vi "Periodic Tasks.vi"(8 "error in":errorcluster) -> ()   [LabVIEW 2013]
doc: "This VI runs in parallel to other tasks. It can contain as many user-defined periodic loops as you need. These can carry out PID or other sorts of timed response."
uses:
  <vilib>/Rock Robotics/WPI/Compressor/WPI_CompressorDevRef.ctl
  <vilib>/Rock Robotics/WPI/DigitalInput/WPI_DigitalInputDevRef.ctl
  <vilib>/Rock Robotics/SystemInterfaces/DIO/FPGA_DIOChannel.ctl
  <vilib>/Rock Robotics/SystemInterfaces/Typedef/FPGA_TypedefDigitalModule.ctl
  <vilib>/Rock Robotics/WPI/Relay/WPI_RelayDevRef.ctl
  <vilib>/Rock Robotics/SystemInterfaces/DIO/FPGA_DIORelayChannel.ctl
  <vilib>/Rock Robotics/WPI/Relay/WPI_RelayDirection.ctl
  <vilib>/Rock Robotics/SystemInterfaces/Utilities/FPGA_UtilitiesLED Source.ctl
  <vilib>/Rock Robotics/SystemInterfaces/Utilities/FPGA_UtilitiesLED State.ctl
  <vilib>/Rock Robotics/WPI/RobotDrive/WPI_RobotDriveGetSetRefNum.vi
  Robot Global Data.vi
  <vilib>/Rock Robotics/WPI/Joystick/WPI_JoystickGetSetRefNum.vi
panel:
  out "output cluster":T1={"DevStatus"={"status"=FALSE, "code"=0, "source"=""}, "DigitalInputDevRef"={"DevStatus"={"status"=FALSE, "code"=0, "source"=""}, "DIO Channel"=enum."DIO 1", "Digital Module"=enum."Digital Module 1"}, "RelayDevRef"={"DevStatus"={"status"=FALSE, "code"=0, "source"=""}, "Relay Channel"=enum."Invalid", "Digital Module"=enum."Digital Module 1", "Relay Direction"=enum."Both directions"}}
  out "Robot Driving":bool
  out "10 ms Counter":i32
  out "100 ms Counter":i32
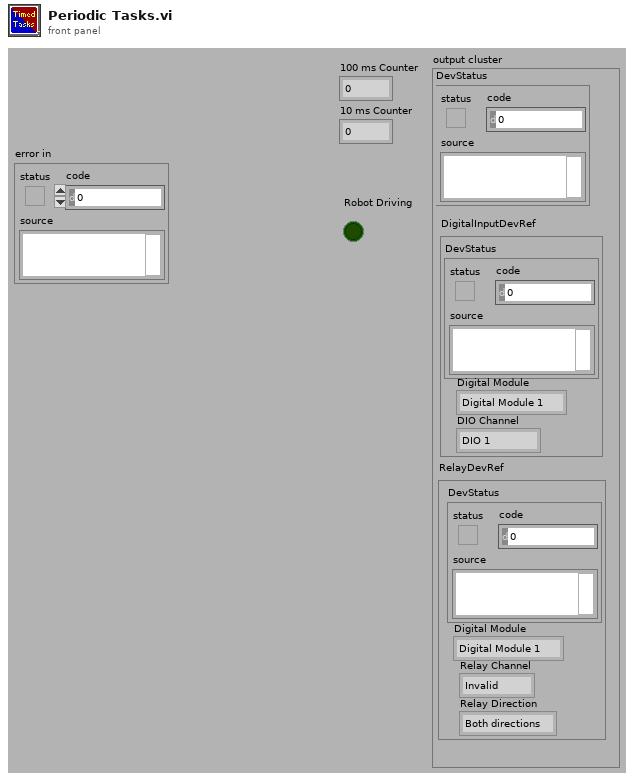
[diagram p1: front panel]
types:
  T1 = typedef "WPI_CompressorDevRef.ctl" = cluster{"DevStatus":errorcluster, "DigitalInputDevRef":T2, "RelayDevRef":T5}
  T2 = typedef "WPI_DigitalInputDevRef.ctl" = cluster{"DevStatus":errorcluster, "DIO Channel":T3, "Digital Module":T4}
  T3 = typedef "FPGA_DIOChannel.ctl" = enum8{"DIO 1", "DIO 2", "DIO 3", "DIO 4", "DIO 5", "DIO 6", "DIO 7", "DIO 8", "DIO 9", "DIO 10", "DIO 11", "DIO 12", "DIO 13", "DIO 14", "Invalid"}
  T4 = typedef "FPGA_TypedefDigitalModule.ctl" = enum16{"Digital Module 1", "Digital Module 2"}
  T5 = typedef "WPI_RelayDevRef.ctl" = cluster{"DevStatus":errorcluster, "Relay Channel":T6, "Digital Module":T4, "Relay Direction":T7}
  T6 = typedef "FPGA_DIORelayChannel.ctl" = enum8{"Relay 1", "Relay 2", "Relay 3", "Relay 4", "Relay 5", "Relay 6", "Relay 7", "Relay 8", "Invalid"}
  T7 = typedef "WPI_RelayDirection.ctl" = enum16{"Both directions", "Forward only", "Reverse only"}
  T8 = typedef "FPGA_UtilitiesLED State.ctl" = enum16{"Off", "On", "Toggle"}
  T9 = typedef "FPGA_UtilitiesLED Source.ctl" = enum16{"User LED", "FPGA LED"}
  T10 = typedef "WPI_JoystickDevRef.ctl" = cluster{"Device":T11}
  T11 = typedef "WPI_JoystickDeviceEnum.ctl" = enum16{"USB 1", "USB 2", "USB 3", "USB 4", "Kinect 1", "Kinect 2"}
  T12 = typedef "WPI_RobotDriveDevRef.ctl" = cluster{"DevStatus":errorcluster, "Motors[]":T13[], "Square Inputs":bool, "Max Output":dbl, "Isochronous":bool}
  T13 = typedef "WPI_MotorControlDeviceRef.ctl" = cluster{"DeviceStatus":errorcluster, "Type":enum16{"PWM", "CAN"}, "PWM":cluster{"Digital Module":T4, "PWM Channel":T14, "DeadBand":T15}, "CAN":cluster{"Device Number":u8, "Control Mode":T16, "Semaphore":T17, "Max Vout":dbl}, "Invert":bool, "TransformRef":T18, "InvTransformRef":T18}
  T14 = typedef "FPGA_DIOPWMChannel.ctl" = enum8{"PWM 1", "PWM 2", "PWM 3", "PWM 4", "PWM 5", "PWM 6", "PWM 7", "PWM 8", "PWM 9", "PWM 10", "Invalid"}
  T15 = typedef "WPI_PWMDeadband.ctl" = cluster{"Name":string, "maxPositivePwm":i32, "minPositivePwm":i32, "centerPwm":i32, "maxNegativePwm":i32, "minNegativePwm":i32, "angularRange":u16}
  T16 = typedef "WPI_CANJaguar_ControlMode.ctl" = enum8{"Percent VBus", "Current", "Speed", "Position", "Voltage"}
  T17 = typedef "Semaphore RefNum" = refnum<k1>
  T18 = typedef "WPI_PWMTransform_ConPane.ctl" = refnum<vi>
  T19 = cluster{"JoystickDevRef":T10, "RobotDriveDevRef":T12}
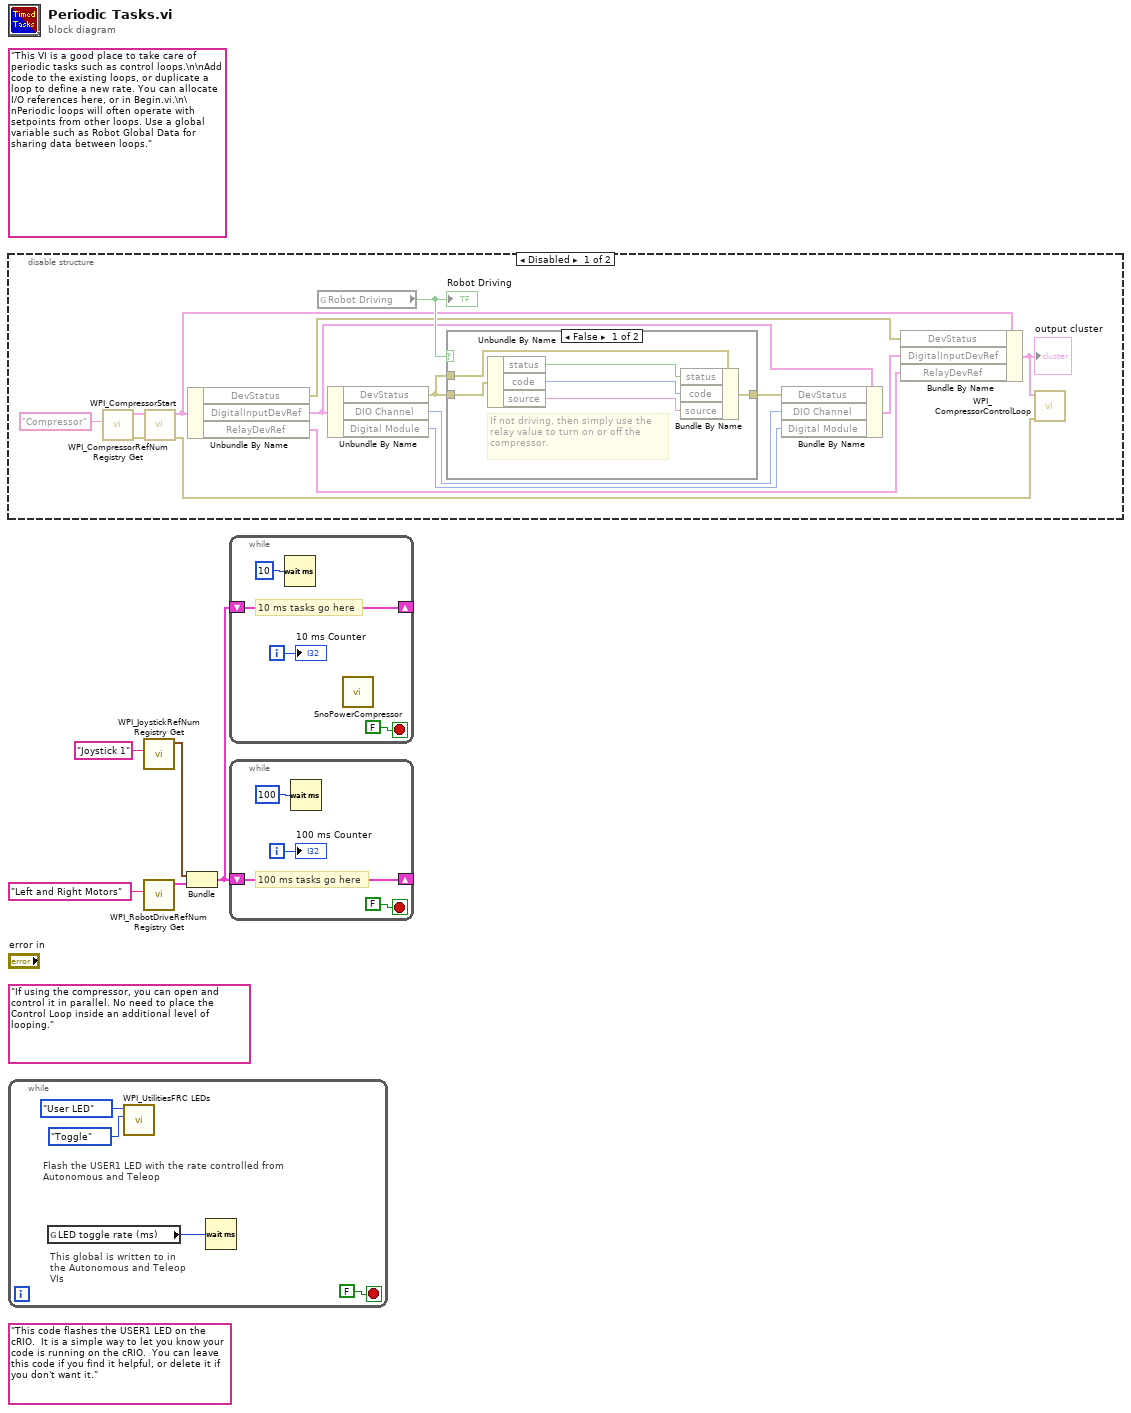
[diagram p0: block diagram]
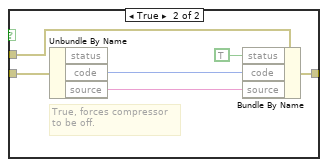
[diagram p2: hidden frame]
diagram:
  (unwired) "If using the compressor, you can open and control it in parallel. No need to place the Control Loop inside an additional level of looping."
  (unwired) "This code flashes the USER1 LED on the cRIO.  It is a simple way to let you know your code is running on the cRIO.  You can leave this code if you find it helpful, or delete it if you don't want it."
  (unwired) "This VI is a good place to take care of periodic tasks such as control loops.\n\nAdd code to the existing loops, or duplicate a loop to define a new rate. You can allocate I/O references here, or in Begin.vi.\n\nPeriodic loops will often operate with setpoints from other loops. Use a global variable such as Robot Global Data for sharing data between loops."
  n1 = disable-structure shown="Disabled" {
    frame Disabled {
      n2 = call <vilib>:"WPI_CompressorRefNum Registry Get.vi"("refnum name"="Compressor") -> ("error out"=w18:errorcluster, "CompressorDevRef"=w19:T1)  [unwired: 9 in]
      n3 = call <vilib>:"WPI_CompressorStart.vi"("error in (no error)"=w18, "CompressorDevRef"=w19) -> ("error out"=w17:errorcluster, "CompressorDevRef"=w12:T1)  [unwired: 8 in]
      n4 = Unbundle By Name(w12) -> ("DevStatus"=w11:errorcluster, "DigitalInputDevRef"=w15:T2, "RelayDevRef"=w10:T5)
      n5 = global read "Robot Global Data.vi" "Robot Driving"() -> (w16:bool)
      "Robot Driving" <- w16
      n6 = Unbundle By Name(w15) -> ("DevStatus"=w7:errorcluster, "DIO Channel"=w14:T3, "Digital Module"=w13:T4)
      n7 = case shown="False" w16 {
        tunnel: [w21 w32] -> w8
        tunnel: w7 -> [w23 w31]
        tunnel: w7 -> [w22 w30]
        frame False {
          # "If not driving, then simply use the\nrelay value to turn on or off the\ncompressor."
          n8 = Unbundle By Name(w22) -> ("status"=w26:bool, "code"=w25:i32, "source"=w24:string)
          n9 = Bundle By Name(cluster=w23, "status"=w26, "code"=w25, "source"=w24) -> (w21:errorcluster)
        }
        frame True {
          # "True, forces compressor\nto be off."
          n10 = Unbundle By Name(w30) -> ("code"=w29:i32, "source"=w28:string)  [unwired: 1 out]
          n11 = Bundle By Name(cluster=w31, "status"=TRUE, "code"=w29, "source"=w28) -> (w32:errorcluster)
        }
      }
      n12 = Bundle By Name(cluster=w15, "DevStatus"=w8, "DIO Channel"=w14, "Digital Module"=w13) -> (w9:T2)
      n13 = Bundle By Name(cluster=w12, "DevStatus"=w11, "DigitalInputDevRef"=w9, "RelayDevRef"=w10) -> (w6:T1)
      "output cluster" <- w6
      n14 = call <vilib>:"WPI_CompressorControlLoop.vi"("error in (no error)"=w17, "CompressorDevRef"=w6) -> ()  [unwired: 10 in]
    }
    frame Enabled {
    }
  }
  n15 = while {
    stop <- FALSE stop-if-true
    # "This global is written to in the Autonomous and Teleop VIs"
    # "Flash the USER1 LED with the rate controlled from Autonomous and Teleop"
    n16 = global read "Robot Global Data.vi" "LED toggle rate (ms)"() -> (w33:u32)
    n17 = call <vilib>:"WPI_UtilitiesFRC LEDs.vi"("State"=FPGA_UtilitiesLED_State."Toggle", "LED Type"=FPGA_UtilitiesLED_Source."User LED") -> ()  [unwired: 1 in, 9 out]
    n18 = Wait (ms)(milliseconds to wait=w33) -> ()  [unwired: 1 out]
  }
  n19 = call <vilib>:"WPI_JoystickRefNum Registry Get.vi"("refnum name"="Joystick 1") -> ("JoystickDevRef"=w3:T10)  [unwired: 1 in, 9 out]
  n20 = call <vilib>:"WPI_RobotDriveRefNum Registry Get.vi"("refnum name"="Left and Right Motors") -> ("RobotDriveDevRef"=w2:T12)  [unwired: 1 in, 9 out]
  n21 = Bundle("JoystickDevRef"=w3, "RobotDriveDevRef"=w2) -> (w1:T19)  [unwired: 1 out]
  n22 = while {
    shift-right: [w38] -> _
    shift-left: w1 -> [w38]
    i -> [w37]
    stop <- FALSE stop-if-true
    # "10 ms tasks go here"
    n23 = Wait (ms)(milliseconds to wait=u32 10) -> ()  [unwired: 1 out]
    n24 = call "SnoPowerCompressor.vi"() -> ()  [unwired: 1 in, 1 out]
    "10 ms Counter" <- w37
  }
  n25 = while {
    shift-right: [w42] -> _
    shift-left: w1 -> [w42]
    i -> [w41]
    stop <- FALSE stop-if-true
    # "100 ms tasks go here"
    n26 = Wait (ms)(milliseconds to wait=u32 100) -> ()  [unwired: 1 out]
    "100 ms Counter" <- w41
  }
